vi "UdsWrite.vi"(5 "LogSuspend":bool, 7 "TimeoutMs":u32=1000, 8 "error in":errorcluster {"code" format="%.0x"}, 9 "DataIn":u8[](array[numeric]) format="%02x", 11 "UdsHandleIn":T1={"LogPath"=path "", "LogEnabled"=FALSE, "isOpen"=FALSE, "LogContent"="", "Adapter"="LIN0", "MCanHandle"={"MCanAdapter"=refnum}, "TransmittId"=0, "ReceiveId"=0}) -> (0 "error out":errorcluster, 3 "UdsHandleOut":T1={"LogPath"=path "", "LogEnabled"=FALSE, "isOpen"=FALSE, "LogContent"="", "Adapter"="LIN0", "MCanHandle"={"MCanAdapter"=refnum}, "TransmittId"=0, "ReceiveId"=0})   [LabVIEW 2011, in "Konvolucio MUDS150628.lvlib"]
uses:
  <instrlib>/Konvolucio MUDS150628/Konvolucio MUDS150628.lvlib
  <instrlib>/Konvolucio MUDS150628/Types/UdsHandleType.ctl
  <instrlib>/Konvolucio MCAN120803/Types/MCanHandleType.ctl
  C:/Program Files/National Instruments/LabVIEW 2011/instr.lib/Konvolucio MCAN120803/Private/Konvolucio.MCAN120803.dll
  Konvolucio MCAN120803/Private/Konvolucio.MCAN120803.dll
  <instrlib>/Konvolucio MCAN120803/Types/MessageType.ctl
  <instrlib>/Konvolucio MUDS150628/Private/UdsLogCanTxMessage.vi
  <instrlib>/Konvolucio MUDS150628/Private/UdsLogErrorCheckPoint.vi
  <instrlib>/Konvolucio MCAN120803/Konvolucio MCAN120803.lvlib
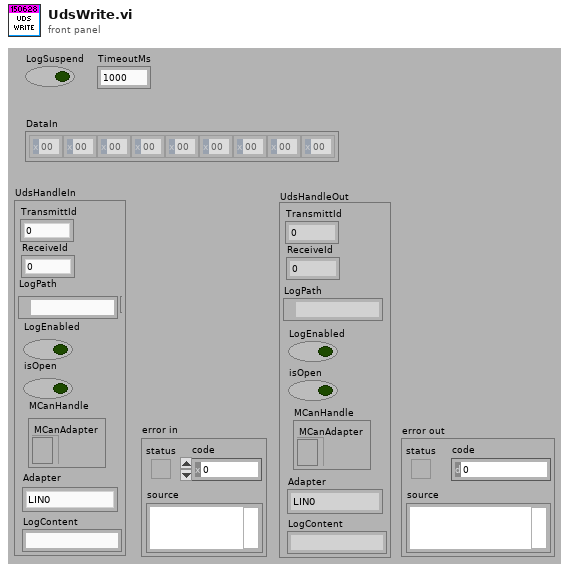
[diagram p1: front panel]
types:
  T1 = typedef "Konvolucio MUDS150628.lvlib/UdsHandleType.ctl" = cluster{"LogPath":path, "LogEnabled":bool, "isOpen":bool, "LogContent":string, "Adapter":string, "MCanHandle":T2, "TransmittId":u32, "ReceiveId":u32}
  T2 = typedef "Konvolucio MCAN120803.lvlib/MCanHandleType.ctl" = cluster{"MCanAdapter":refnum<k24>}
  T3 = typedef "Konvolucio MCAN120803.lvlib/MessageType.ctl" = cluster{"TimeStamp":timestamp, "ArbitrationId":u32, "IsRemote":u8, "DataLength":u8, "Data":u8[]}
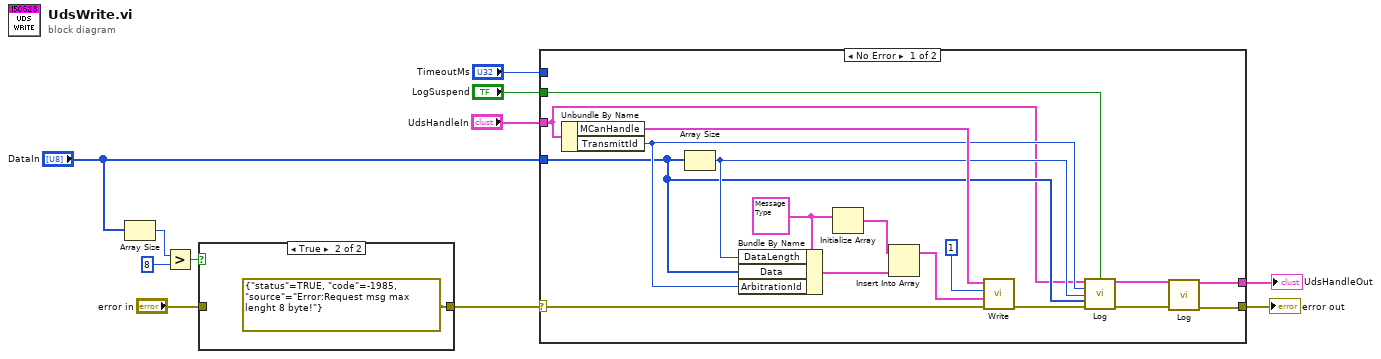
[diagram p0: block diagram]
diagram:
  n1 = Array Size(array="DataIn") -> (size(s)=w10:i32)
  n2 = Greater?(x=w10, y=8) -> (0:w7:bool)
  n3 = case shown="True" w7 {
    tunnel: [w12 errorcluster {"status"=TRUE, "code"=-1985, "source"="Error:Request msg max lenght 8 byte!"} ("error in")] -> w6
    tunnel: "error in" -> [w12 _]
    frame False {
    }
    frame True {
    }
  }
  n4 = case shown="No Error" w6 {
    selector: w6 -> [w24 w32]
    tunnel: "DataIn" -> [w20 _]
    tunnel: [w14 w32] -> w11
    tunnel: "UdsHandleIn" -> [w19 w31]
    tunnel: [w15 w31] -> w3
    tunnel: "TimeoutMs" -> [_ _]
    tunnel: "LogSuspend" -> [w18 _]
    frame No Error {
      w26 = T3 {"TimeStamp"=timestamp(0 s since 1904-01-01), "ArbitrationId"=0, "IsRemote"=0, "DataLength"=0, "Data"=[]}
      n5 = Unbundle By Name(w19) -> ("MCanHandle"=w29:T2, "TransmittId"=w22:u32)
      n6 = Array Size(array=w20) -> (size(s)=w21:i32)
      n7 = Bundle By Name(cluster=w26, "DataLength"=w21, "Data"=w20, "ArbitrationId"=w22) -> (w25:T3)
      n8 = Initialize Array(w26) -> (w28:T3[])  [unwired: 1 in]
      n9 = Insert Into Array(array=w28, new element=w25) -> (w27:T3[])  [unwired: 1 in]
      n10 = call <instrlib>:"Write.vi"("error in"=w24, "Messages"=w27, "Number to Write"=1, "MCanHandleIn"=w29) -> ("error out"=w23:errorcluster)  [unwired: 4 in, 1 out]
      n11 = call-poly <instrlib>:"Log.vi"("UdsHandleIn"=w19, "LogSuspend"=w18, "Id"=w22, "DataLength"=w21, "Data"=w20, "error in"=w23) -> ("UdsHandleOut"=w17:T1, "error out"=w16:errorcluster)  [unwired: 8 in]
      n12 = call-poly <instrlib>:"Log.vi"("UdsHandleIn"=w17, "error in"=w16) -> ("UdsHandleOut"=w15:T1, "error out"=w14:errorcluster)  [unwired: 12 in]
    }
    frame Error {
    }
  }
  "error out" <- w11
  "UdsHandleOut" <- w3
